vi "Testing Mode.vi"(8 "Filepath":path=path "D:/My Project/2019-2020/Magnetic Mareli UM/MM_UM/Project Setup/data/program seq/Program_280A.bin", 9 "FeedBack Channel":string[](array[string])=["fgdgfvcbc", "vnfhgjkn", "21354682"]) -> ()   [LabVIEW 2015]
uses:
  Control Button/Exit.ctl
  Control Button/Start.ctl
  Test  enqueue/AutoTest seq.ctl
  Test  enqueue/Auot Test selection.ctl
  <vilib>/Utility/error.llb/whitespace.ctl
  Galobal variable_TI.vi
  Project Setup/Globle Variable/GR_Servo.vi
  <vilib>/Utility/file.llb/Read Delimited Spreadsheet (string).vi
panel:
  out "Error  bit":bool
  out "reset":bool
  out "D-enqueue":T1
  in  "Report":bool
  in  "Tab Control":enum32{"Test", "Report"}(tab)
  in  "Boolean":bool=TRUE
  out "User Name":string
  in  "Table Control":string[][](table)
  out "Error Message":string
  out "Running Model":string
  out "Date time":string
  out "PCB Barcode":string
  out "Test Name":string
  in  "Tab Control 2":enum32{"Image", "Load and Lvdt"}(tab)
  out "2D Picture":picture
  out "Boolean 3":bool
  out "Waveform Graph":dbl[](graph)
  out "Error":bool
  in  "Exit":T2
  in  "Start 2":T3
  in  "Slide Servo Home Call":bool
  out "Servo Fault":bool
  in  "Servo Fault Reset":bool
  out "Actuator2(mm)":dbl format="%0.02f"
  out "Actuator1(mm)":dbl format="%0.02f"
  out "Load(N)":dbl format="%0.02f"
  out "Clip":T4
  in  "OK Counter":string
  in  "NG Counter":string
  out "Cycle Time(Sec)":i32
  out "Camera Result":bool
  in  "Report":i32(listbox)
  out "appended array":string[](array[string])
  in  "Sensor Feedback":T5(array[cluster])
  out "Start":bool
  in  "Cycle":i32
  in  "Home Call":bool
  out "DI":bool[](array[boolean])
  out "Current Date & Time":timestamp
  in  "Cycle Start Bit":bool
  in  "vi reference":refnum<vi>
  in  "Reset Ct.":bool
  out "error out":errorcluster
  in  "Tbl Refnum":refnum<vi>
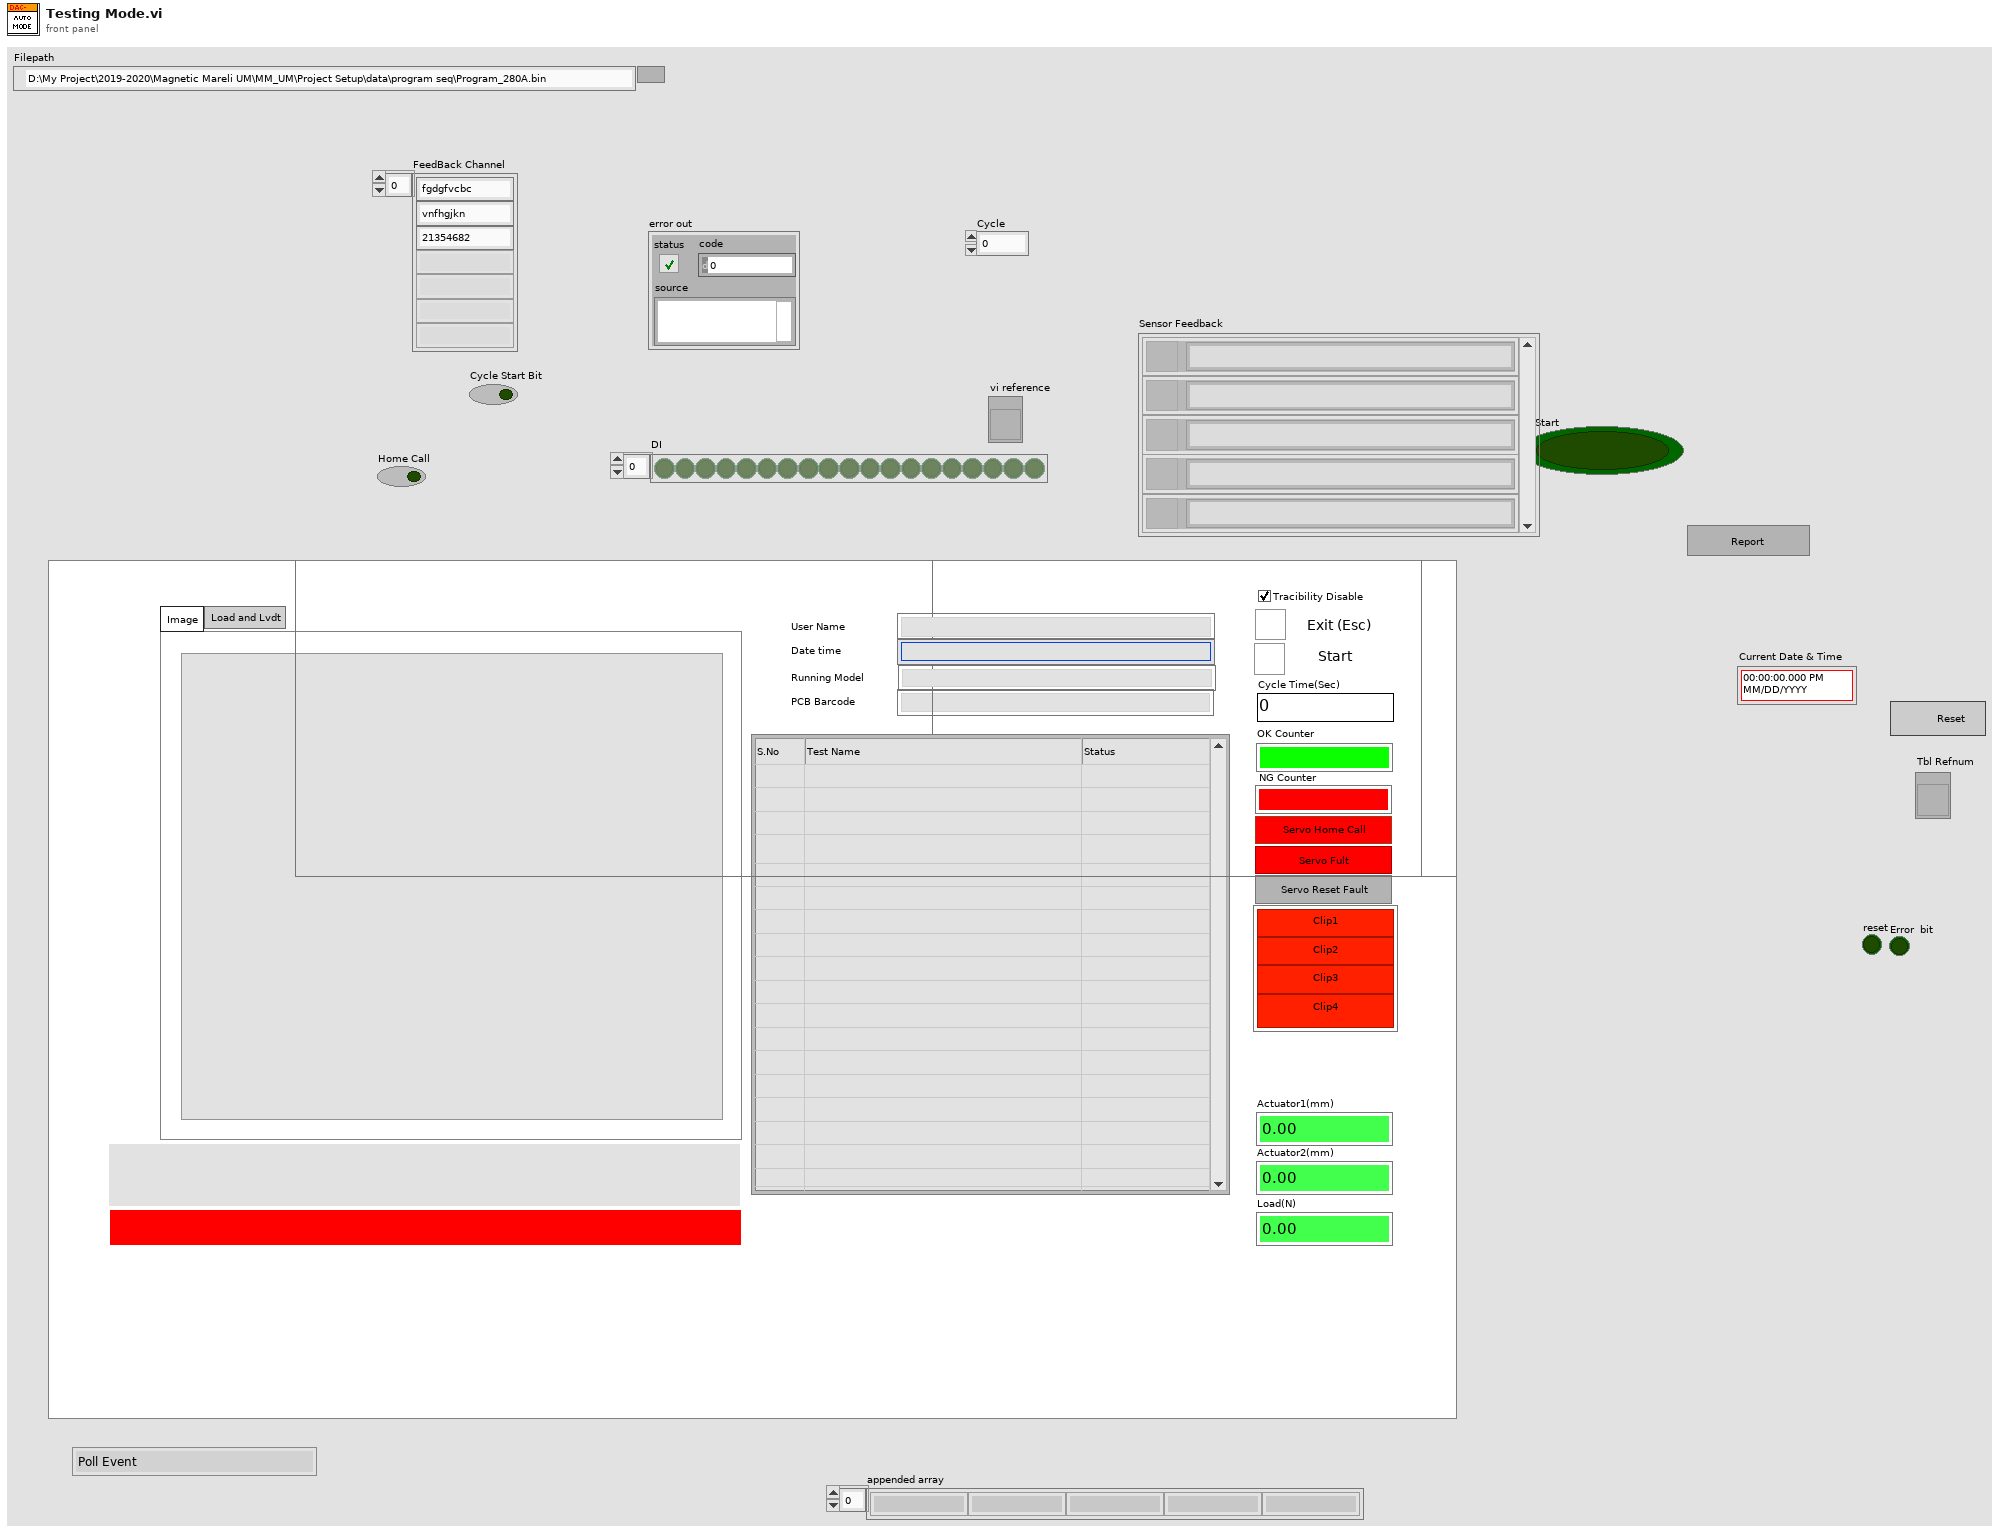
[diagram p1: front panel]
types:
  T1 = typedef "AutoTest seq.ctl" = enum16{"Poll Event", "Fixture 40 Deg up", "Program Seq", "Cylender Home", "Read Barcode", "Slide Servo send Cammand", "Slide Servo Home Call", "Camera Co-ordinate_1", "Camera Co-ordinate_2", "Result Save", "Error", "Exit"}
  T2 = typedef "Exit.ctl" = bool
  T3 = typedef "Start.ctl" = bool
  T4 = cluster{"Cllip-3 (AI12)":bool, "Cllip-4 (AI9)":bool, "Cllip-2(AI10)":bool, "Cllip-1 (AI9)":bool}
  T5 = cluster{"Sensor Name":string, "OK And NG":bool}[]
  T6 = cluster{"MIC ":refnum<visa-resource-name>, "baud rate MIC ":u32, "LCD ":refnum<visa-resource-name>, "baud rate_LCD":u32}
  T7 = typedef "Auot Test selection.ctl" = enum16{"Init", "Enqueue ", "Enqueue N", "Enqueue in stack", "Enqueue in stack N", "Dequeue", "Dequeue N", "Flush", "Release Queue"}
  T8 = cluster{"Item Name":string, "Item Status":bool, "Steps":cluster{"Channel Type":string, "Channels":string, "Wait/Poll (ms)":u32, "Parameter":u8, "STM-Speed":i32, "STM-Degree":u32, "Direction":u8}[]}[]
  T9 = cluster{"Actuator1(mm)":dbl, "Actuator2(mm)":dbl, "Load(N)":dbl, "Actuator1":bool, "Actuator2":bool, "Load":bool}
  T10 = enum16{"Part Clamp", "Part Unclamp", "Part Clamp Input Check", "Part Unclamp Input Check"}
  T11 = cluster{"Sr.No.":string, "Model Pass/Fail":string, "MIC Code":string, "Clip-1":string, "Clip-2":string, "Clip-3":string, "Clip-4":string, "Load Max":string, "Load Min":string, "Load Actual Value":string, "Actuator -1Min":string, "Actuator -1Max":string, "Actuator-1 Actual Value":string, "Actuator -2Min ":string, "Actuator -2Max ":string, "Actuator-2 Actual Value ":string, "Status":string}
  T12 = cluster{"No. Fail Coun t":string, "Rework Status Count 0\\1":string, "NA Count Max =3 ":string, "Testesd Count  0/1":string, "Error code":string}
  T13 = cluster{"Emergency_1":bool, "Reset_2":bool, "Home _3":bool, "Air Pressure_4":bool, "Safety Sensor_5":bool, "Safety Sensor_6":bool, "Slide Servo Home RS 26":bool, "LVDT UP RS":bool, "Servo Fault 27":bool, "Pressing UP RS 31":bool, "40 Deg. Down Fixture Rs":bool}
  T14 = typedef "whitespace.ctl" = u16
  T15 = cluster{"Load Max":string, "Load Min":string, "Actuator -1 Max":string, "Actuator -1 Min":string, "Actuator -2 Max":string, "Actuator -2 Min":string}
  T16 = cluster{"Sr.No.":string, "Model Name":string, "Date":string, "Time":string, "Model Pass/Fail":string, "MIC Code":string, "Clip-1":string, "Clip-2":string, "Clip-3":string, "Clip-4":string, "Load Max":string, "Load Min":string, "Load Actual Value":string, "Actuator -1Min":string, "Actuator -1Max":string, "Actuator-1 Actual Value":string, "Actuator -2Min ":string, "Actuator -2Max ":string, "Actuator-2 Actual Value ":string, "Status":string}
  T17 = cluster{"[0]":string, "[1]":string, "[2]":string, "[3]":string}
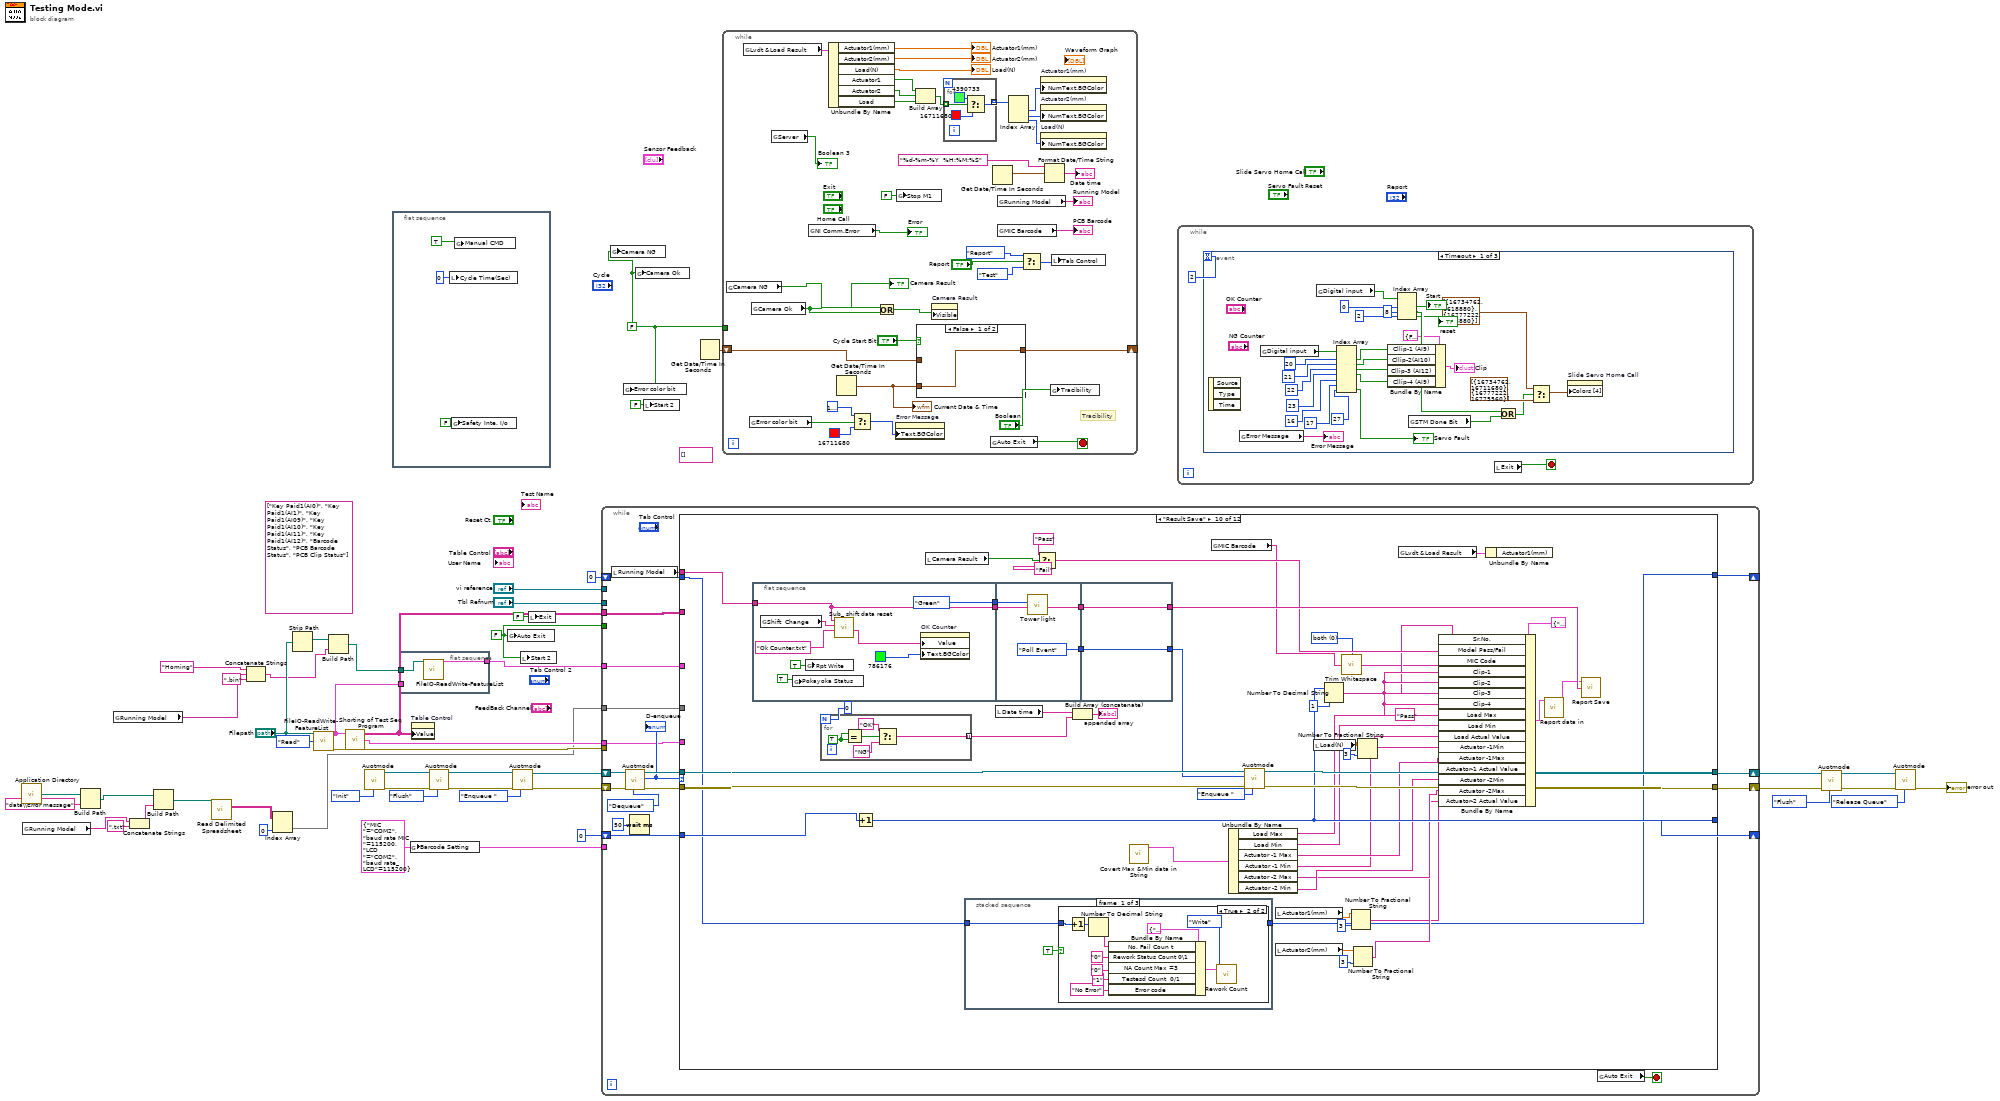
[diagram p0: block diagram]
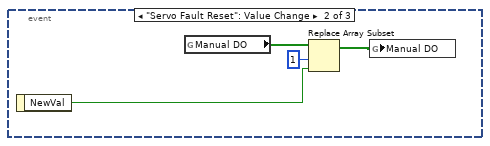
[diagram p2: hidden frame]
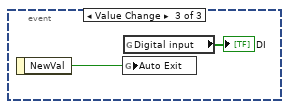
[diagram p3: hidden frame]
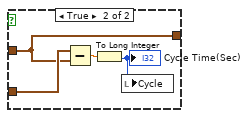
[diagram p4: hidden frame]
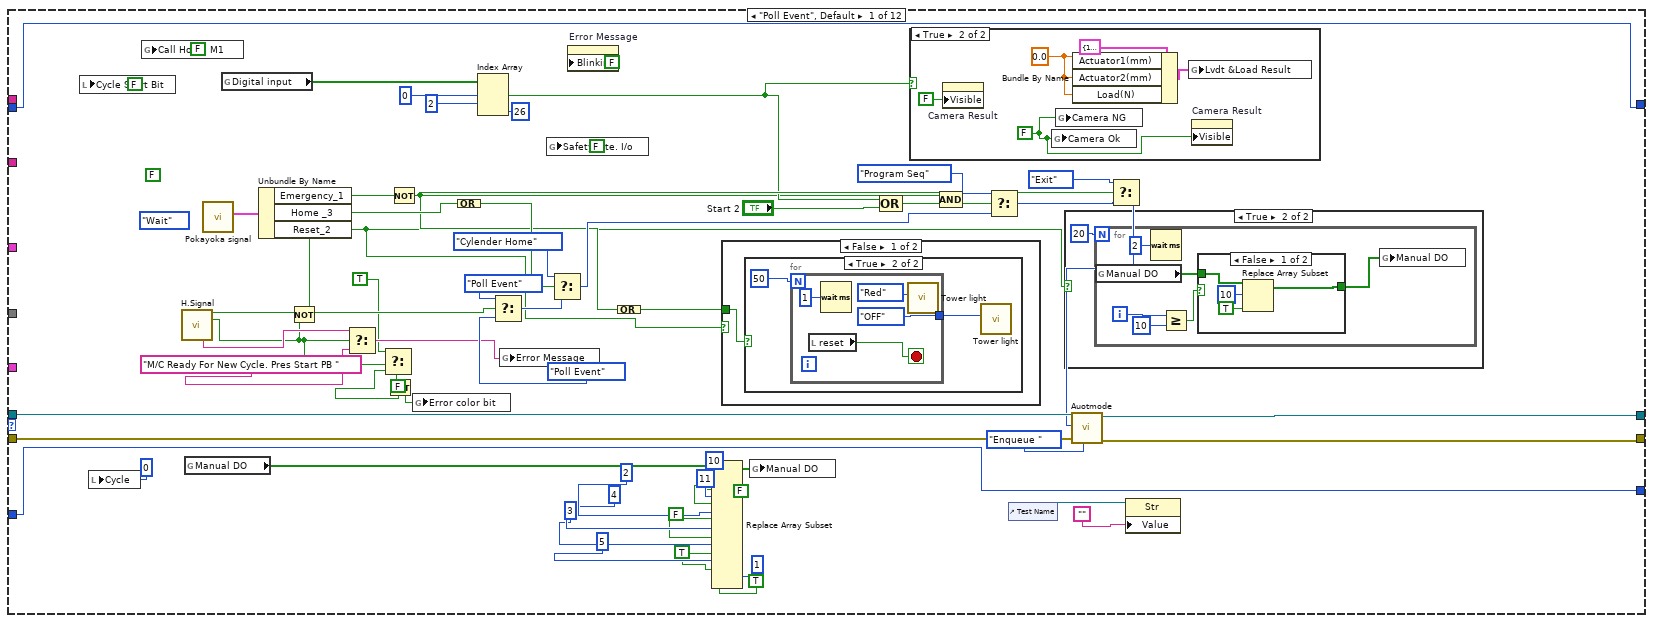
[diagram p5: hidden frame]
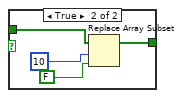
[diagram p7: hidden frame]
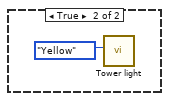
[diagram p10: hidden frame]
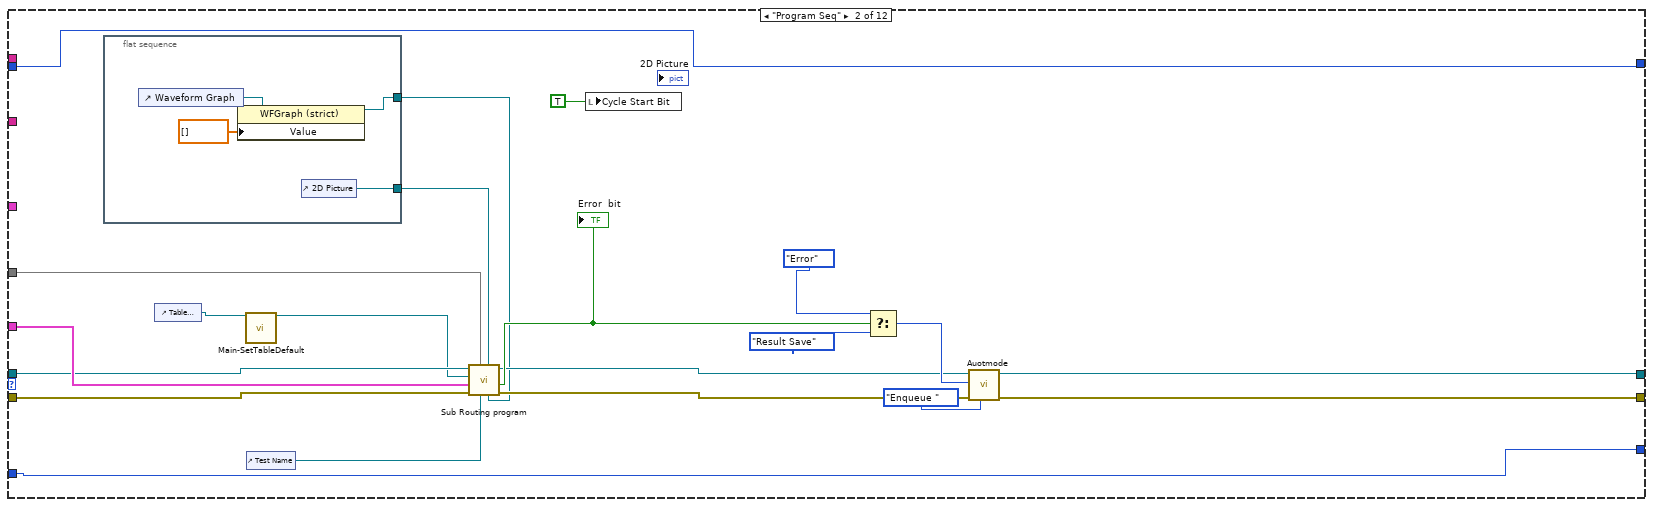
[diagram p11: hidden frame]
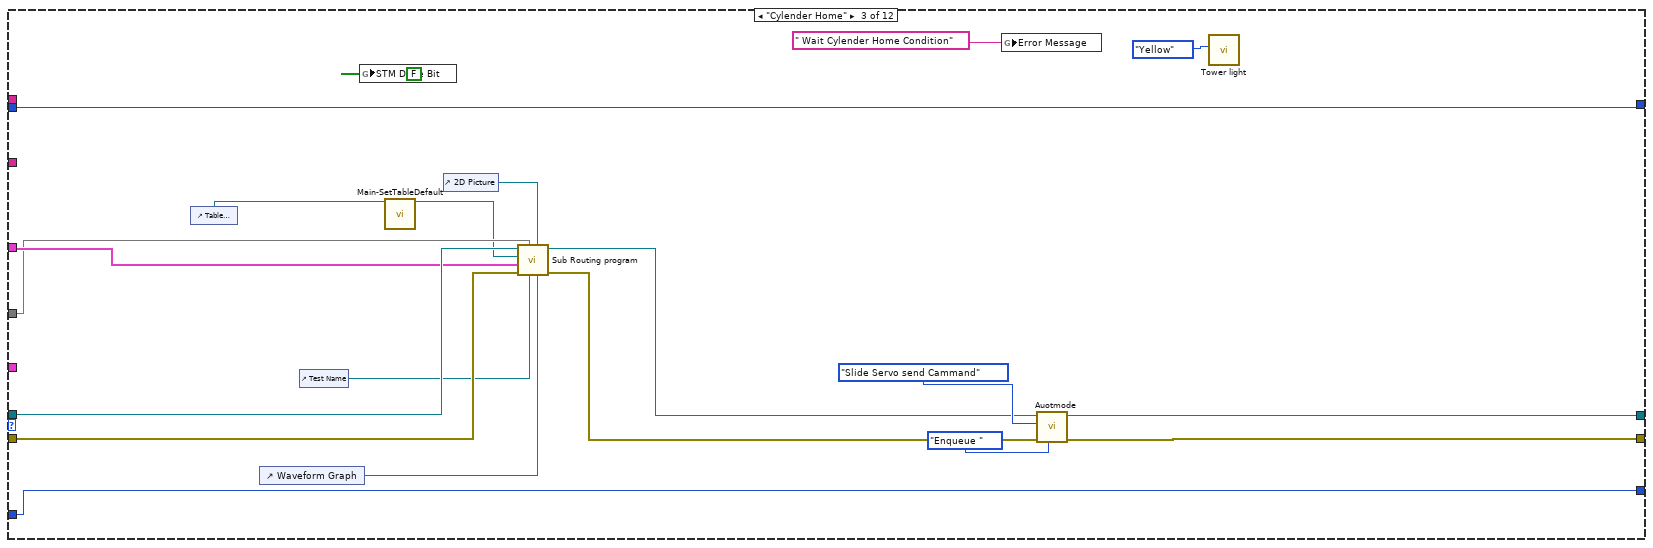
[diagram p12: hidden frame]
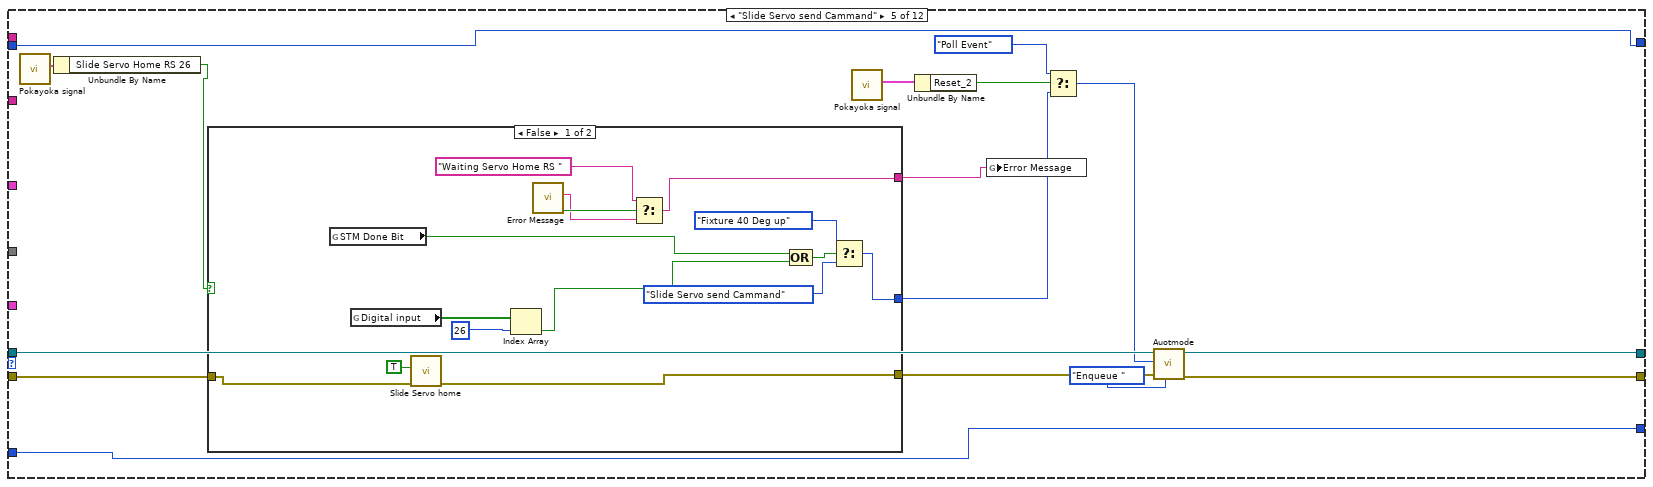
[diagram p14: hidden frame]
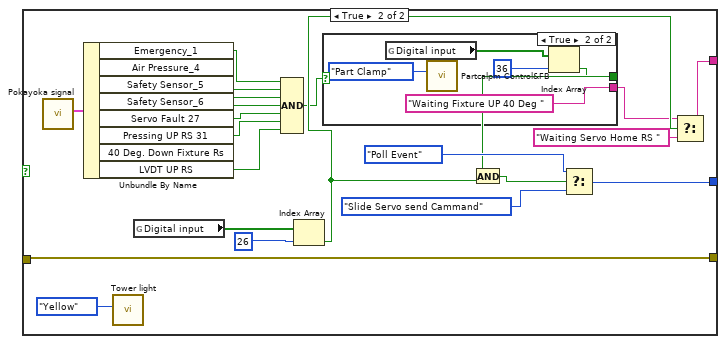
[diagram p15: hidden frame]
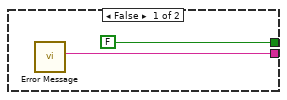
[diagram p16: hidden frame]
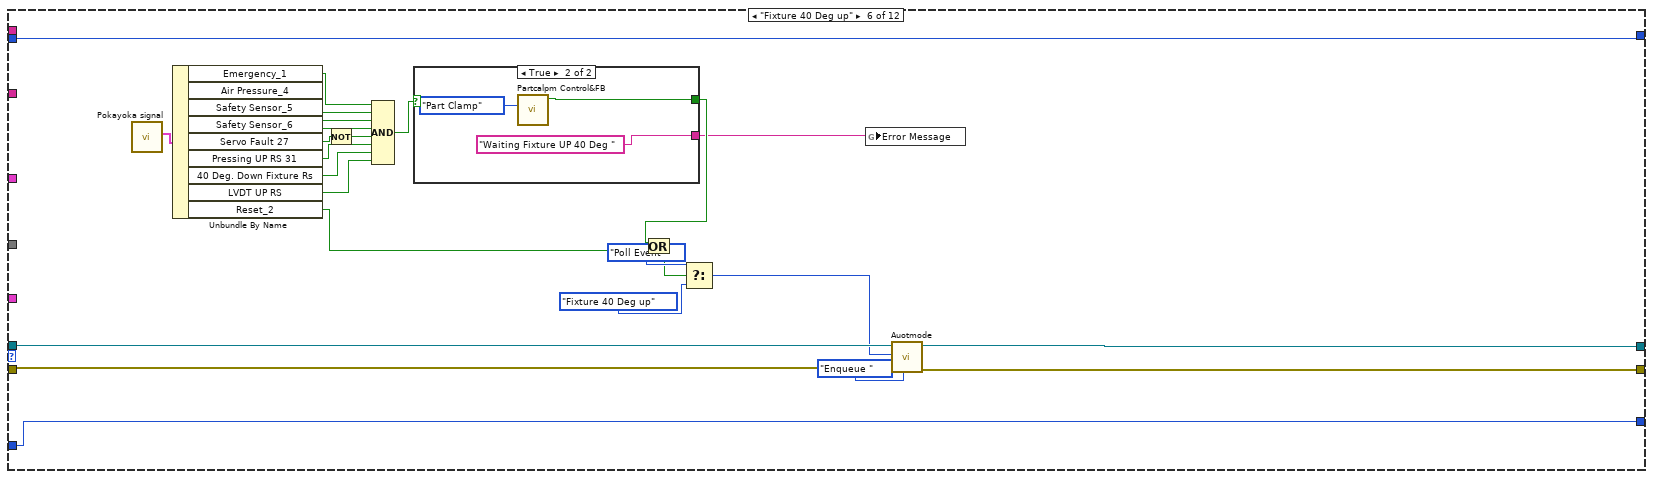
[diagram p17: hidden frame]
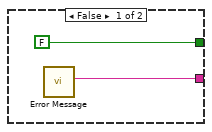
[diagram p18: hidden frame]
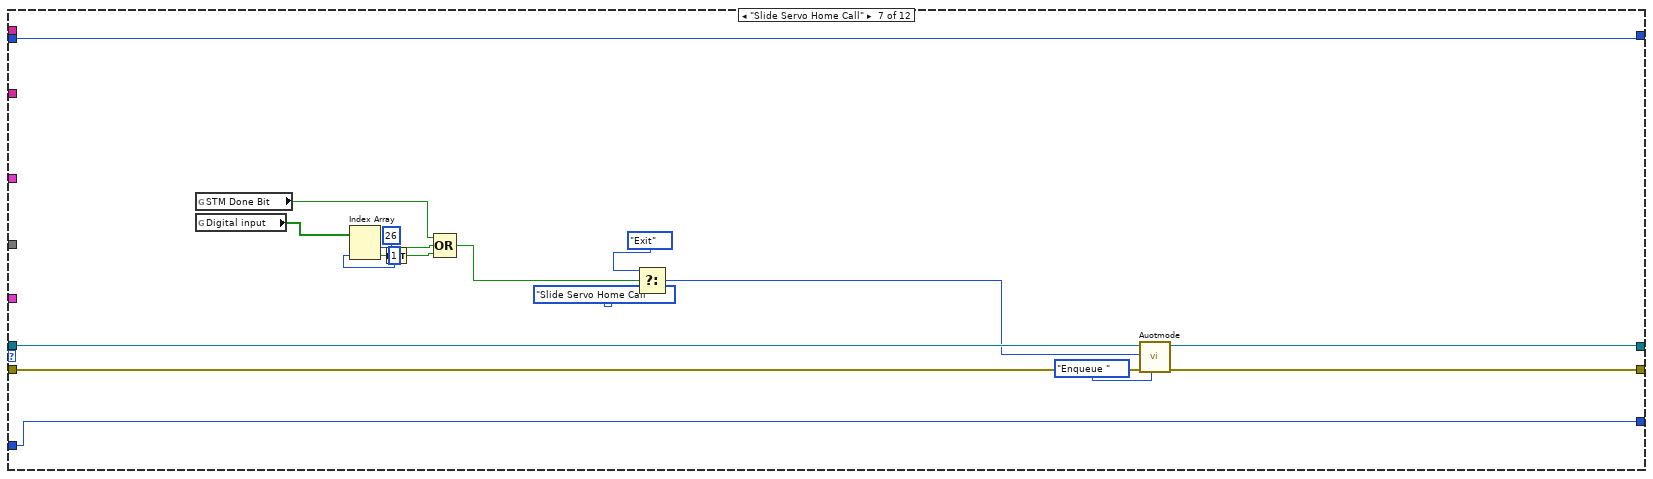
[diagram p19: hidden frame]
diagram:
  w18 = T6 {"MIC "="COM2", "baud rate MIC "=115200, "LCD "="COM2", "baud rate_LCD"=115200} ("Barcode Setting")
  (unwired) string[] ["Key Paid1(AI0)", "Key Paid1(AI1)", "Key Paid1(AI09)", "Key Paid1(AI10)", "Key Paid1(AI11)", "Key Paid1(AI12)", "Barcode Status", "PCB Barcode Status", "PCB Clip Status"] ("Error Name")
  (unwired) string[] []
  w3 = FALSE ("Servo Stop")
  w25 = FALSE ("Auto Exit")
  n1 = call <vilib>:"Application Directory.vi"() -> ("Application Directory"=w17:path)
  n2 = global read "Galobal variable_TI.vi" "Running Model"() -> (w14:string)
  n3 = Build Path(base path=w17, name or relative path="data\\Error message") -> (appended path=w15:path)
  n4 = global read "Galobal variable_TI.vi" "Running Model"() -> (w6:string)
  n5 = Concatenate Strings(w14, ".txt" ("string")) -> (w12:string)
  n6 = Build Path(base path=w15, name or relative path=w12) -> (appended path=w11:path)
  n7 = call-poly <vilib>:"Read Delimited Spreadsheet.vi"("file path (dialog if empty)"=w11) -> ("all rows"=w10:string[][])  [unwired: 9 in, 5 out]
  n8 = Concatenate Strings("Homing" ("name or relative path"), w6, ".bin" ("string")) -> (w4:string)
  n9 = Index Array(array=w10, index (col)=0 ("disabled index (col)")) -> (element=w8:string[])  [unwired: 1 in]
  n10 = Strip Path(path="Filepath") -> (stripped path=w22:path)  [unwired: 1 out]
  n11 = call "FileIO-ReadWrite-FeatureList.vi"("Filepath"="Filepath", "Read/Write"=enum16{"Read", "Write"}."Read") -> ("Feature List (Out)"=w20:T8, "Error Out"=w31:errorcluster)  [unwired: 12 in]
  n12 = Build Path(base path=w22, name or relative path=w4) -> (appended path=w21:path)
  n13 = call "Shorting of Test Seq Program.vi"("Feature List (Out)"=w20) -> ("Feature Step Enable"=w27:T8, "Feature Name"=w26:string[][])  [unwired: 3 in]
  n14 = call "Auotmode.vi"("Enum Selection"=Auot_Test_selection."Init") -> ("error out"=w43:errorcluster, "queue Out"=w41:refnum<queue>)  [unwired: 7 in, 1 out]
  n15 = flat-sequence {
    frame #0 {
      n16 = local write "Cycle Time(Sec)"(0 ("Cycle Time(Sec)")) -> ()
      n17 = global write "Galobal variable_TI.vi" "Safety Inte. I/o"(FALSE ("Safety Inte. I/o")) -> ()
      n18 = global write "Galobal variable_TI.vi" "Manual CMD"(TRUE ("Manual CMD")) -> ()
    }
  }
  n19 = flat-sequence {
    tunnel: w21 -> [w54]
    tunnel: w20 -> [_]
    tunnel: [w53] -> w19
    frame #0 {
      n20 = call "FileIO-ReadWrite-FeatureList.vi"("Filepath"=w54) -> ("Feature List (Out)"=w53:T8)  [unwired: 13 in, 1 out]
    }
  }
  n21 = global write "Galobal variable_TI.vi" "Barcode Setting"(w18) -> ()
  n22 = property on="Table Control" class="Tbl (strict)"("Value"=w26) -> ()  [unwired: 2 in, 2 out]
  n23 = call "Auotmode.vi"("Enum Selection"=Auot_Test_selection."Flush", "Error In"=w43, "queue in"=w41) -> ("error out"=w42:errorcluster, "queue Out"=w40:refnum<queue>)  [unwired: 5 in, 1 out]
  n24 = global write "Galobal variable_TI.vi" "Auto Exit"(w25) -> ()
  n25 = call "Auotmode.vi"("Enum Selection"=Auot_Test_selection."Enqueue ", "Error In"=w42, "queue in"=w40) -> ("error out"=w47:errorcluster, "queue Out"=w29:refnum<queue>)  [unwired: 5 in, 1 out]
  n26 = local write "Start 2"(w25) -> ()
  n27 = local write "Exit"(T2 FALSE ("Exit")) -> ()
  n28 = while {
    tunnel: "vi reference" -> [_]
    tunnel: "Tbl Refnum" -> [_]
    tunnel: w27 -> [w66]
    tunnel: w31 -> [_]
    tunnel: w8 -> [w67]
    shift-right: [w70] -> w34
    shift-left: w29 -> [w63]
    shift-right: [w62] -> w28
    shift-left: w47 -> [w72]
    tunnel: w25 -> [_]
    tunnel: w26 -> [w61]
    tunnel: w19 -> [w59]
    tunnel: w18 -> [_]
    shift-right: [w57] -> _
    shift-left: u32 0 ("milliseconds to wait") -> [w58]
    shift-right: [w55] -> _
    shift-left: u32 0 ("milliseconds to wait") -> [w56]
    stop <- w65 stop-if-true
    n29 = local read "Running Model"() -> (w60:string)
    n30 = call "Auotmode.vi"("Enum Selection"=Auot_Test_selection."Dequeue", "Error In"=w72, "queue in"=w63) -> ("error out"=w69:errorcluster, "D-enqueue"=w68:T1, "queue Out"=w71:refnum<queue>)  [unwired: 5 in]
    "D-enqueue" <- w68
    n31 = Wait (ms)(milliseconds to wait=u32 50) -> ()  [unwired: 1 out]
    n32 = case shown="\"Result Save\"" w68 {
      tunnel: w71 -> [w134 w172 w204 w211 w222 w284 w316 w323 w327 w376 w432 w544]
      tunnel: [w132 w179 w206 w211 w226 w283 w317 w323 w327 w374 w431 w545] -> w70
      tunnel: w69 -> [w133 w174 w203 w210 w224 w282 w315 w322 w326 w375 w430 w546]
      tunnel: [w131 w178 w205 w210 w225 w281 w318 w322 w326 w373 w429 w546] -> w62
      tunnel: w66 -> [_ w175 _ _ _ _ _ _ _ _ _ _]
      tunnel: w67 -> [_ w176 w201 _ _ _ _ _ _ _ _ _]
      tunnel: w61 -> [_ _ _ _ _ _ _ _ _ _ _ _]
      tunnel: w60 -> [_ _ _ _ _ _ _ _ _ w372 w416 _]
      tunnel: w59 -> [_ _ w202 _ _ _ _ _ _ _ _ _]
      tunnel: w58 -> [w75 w164 w189 w209 w213 w273 w303 w321 w325 w355 w415 w530]
      tunnel: [w75 w164 w189 w209 w213 w273 w303 w321 w325 w354 w415 w530] -> w57
      tunnel: w56 -> [w74 w163 w188 w208 w212 w272 w302 w320 w324 w329 w412 w529]
      tunnel: [w74 w163 w188 w208 w212 w272 w302 w320 w324 w328 w411 w529] -> w55
      frame "Poll Event", Default {
        w79 = TRUE ("new element/subarray")
        w80 = FALSE ("new element/subarray")
        w98 = FALSE ("new element/subarray")
        (unwired) enum16{"Wait", "Ionizer On", "Ionizer off"}."Wait" ("Enum")
        (unwired) FALSE ("Ionizer cnf")
        n33 = local write "Cycle Start Bit"(FALSE ("Cycle Start Bit")) -> ()
        n34 = local write "Cycle"(0 ("Cycle")) -> ()
        n35 = global write "Galobal variable_TI.vi" "Call Home M1"(FALSE ("Call Home M1")) -> ()
        n36 = call "H.Signal.vi"() -> ("Slide servo home RS"=w119:bool, "HI Bit Auto"=w88:bool, "Message"=w95:string)  [unwired: 10 in, 3 out]
        n37 = global read "Galobal variable_TI.vi" "Manual DO"() -> (w86:bool[])
        n38 = call "Pokayoka signal.vi"() -> ("output cluster"=w113:T13)  [unwired: 10 in, 1 out]
        n39 = global read "Galobal variable_TI.vi" "Digital input"() -> (w129:bool[])
        n40 = Unbundle By Name(w113) -> ("Emergency_1"=w112:bool, "Home _3"=w103:bool, "Reset_2"=w96:bool)
        n41 = Not(x=w88) -> (.not. x?=w87:bool)
        n42 = Select(t=w95, s=w88, f="M/C Ready For New Cycle. Pres Start PB ") -> (s? t:f=w108:string)
        n43 = Select(t=TRUE, s=w88, f=FALSE) -> (s? t:f=w92:bool)
        n44 = Not(x=w92) -> (.not. x?=w91:bool)
        n45 = Not(x=w112) -> (.not. x?=w102:bool)
        n46 = global write "Galobal variable_TI.vi" "Error color bit"(w91) -> ()
        n47 = Compound Arithmetic op=OR(w103) -> (w125:bool)
        n48 = Index Array(array=w129, index #1=0 ("index"), index #2=2 ("index"), index #3=26 ("index")) -> (element #1=w97:bool)  [unwired: 2 out]
        n49 = Select(t=AutoTest_seq."Poll Event" ("Enqueue"), s=w119, f=AutoTest_seq."Poll Event") -> (s? t:f=w123:T1)
        n50 = global write "GR_Servo.vi" "Error Message"(w108) -> ()
        n51 = global write "Galobal variable_TI.vi" "Safety Inte. I/o"(FALSE ("Safety Inte. I/o")) -> ()
        n52 = Select(t=AutoTest_seq."Cylender Home" ("Enqueue"), s=w125, f=w123) -> (s? t:f=w111:T1)
        n53 = property on="Error Message" class="Str"("Blinking"=FALSE) -> ()  [unwired: 2 in, 2 out]
        n54 = Compound Arithmetic op=OR(w102) -> (w107:bool)
        n55 = Replace Array Subset(array=w86, new element #1=w98, index #1=10 ("index"), new element #2=w98, index #2=11 ("index"), new element #3=w80, index #3=2 ("index"), new element #4=w80, index #4=4 ("index"), new element #5=w79, index #5=3 ("index"), new element #6=w79, index #6=5 ("index"), new element #7=TRUE ("new element/subarray"), index #7=1 ("index")) -> (w101:bool[])
        n56 = case shown="False" w96 {
          tunnel: w107 -> [w155 _]
          frame False {
            n57 = case shown="True" w155 {
              frame False {
              }
              frame True {
                n58 = for {
                  N: 50 -> [_]
                  tunnel: [enum16{"Green", "Red", "Yellow", "OFF"}."OFF" ("Enum")] -> w156
                  stop <- w158 stop-if-true
                  n59 = local read "reset"() -> (w158:bool)
                  n60 = Wait (ms)(milliseconds to wait=u32 1) -> ()  [unwired: 1 out]
                  n61 = call "Tower light.vi"("Enum"=enum16{"Green", "Red", "Yellow"}."Red") -> ()  [unwired: 11 in]
                }
                n62 = call "Tower light.vi"("Enum"=w156) -> ()  [unwired: 11 in]
              }
            }
          }
          frame True {
            n63 = call "Tower light.vi"("Enum"=enum16{"Green", "Red", "Yellow"}."Yellow") -> ()  [unwired: 11 in]
          }
        }
        n64 = global write "Galobal variable_TI.vi" "Manual DO"(w101) -> ()
        n65 = Compound Arithmetic op=OR(w97, "Start 2") -> (w117:T3)
        n66 = case shown="True" w97 {
          frame False {
          }
          frame True {
            w150 = 0.0
            w153 = FALSE
            n67 = property on="Camera Result" class="Bool (strict)"("Visible"=FALSE) -> ()  [unwired: 2 in, 2 out]
            n68 = global write "Galobal variable_TI.vi" "Camera Ok"(w153) -> ()
            n69 = global write "Galobal variable_TI.vi" "Camera NG"(w153) -> ()
            n70 = Bundle By Name(cluster=T9 {"Actuator1(mm)"=1.6341840742039335, "Actuator2(mm)"=1.8426400447473008, "Load(N)"=41.278042038610465, "Actuator1"=TRUE, "Actuator2"=TRUE, "Load"=TRUE} ("Lvdt &Load Result"), "Actuator1(mm)"=w150, "Actuator2(mm)"=w150, "Load(N)"=w150) -> (w151:T9)
            n71 = global write "Galobal variable_TI.vi" "Lvdt &Load Result"(w151) -> ()
            n72 = property on="Camera Result" class="Bool (strict)"("Visible"=w153) -> ()  [unwired: 2 in, 2 out]
          }
        }
        n73 = Compound Arithmetic op=AND(w87, w117) -> (w89:T3)
        n74 = Select(t=AutoTest_seq."Program Seq" ("Enqueue"), s=w89, f=w111) -> (s? t:f=w105:T1)
        n75 = control-ref of="Test Name"() -> (w110:refnum<vi>)
        n76 = case shown="True" w96 {
          frame False {
          }
          frame True {
            n77 = for {
              N: 20 -> [_]
              i -> [w141]
              n78 = global read "Galobal variable_TI.vi" "Manual DO"() -> (w138:bool[])
              n79 = Wait (ms)(milliseconds to wait=u32 2) -> ()  [unwired: 1 out]
              n80 = Greater Or Equal?(x=w141, y=10) -> (x >= y?=w139:bool)
              n81 = case shown="False" w139 {
                tunnel: w138 -> [w145 w147]
                tunnel: [w142 w146] -> w137
                frame False {
                  n82 = Replace Array Subset(array=w145, new element=TRUE ("new element/subarray"), index=10) -> (w142:bool[])
                }
                frame True {
                  n83 = Replace Array Subset(array=w147, new element=FALSE ("new element/subarray"), index=10) -> (w146:bool[])
                }
              }
              n84 = global write "Galobal variable_TI.vi" "Manual DO"(w137) -> ()
            }
          }
        }
        n85 = Select(t=AutoTest_seq."Exit" ("Enqueue"), s=w102, f=w105) -> (s? t:f=w106:T1)
        n86 = call "Auotmode.vi"("Enum Selection"=Auot_Test_selection."Enqueue ", "Error In"=w133, "Enqueue"=w106, "queue in"=w134) -> ("error out"=w131:errorcluster, "queue Out"=w132:refnum<queue>)  [unwired: 4 in, 1 out]
        n87 = property class="Str"(reference=w110, "Value"="") -> ()  [unwired: 1 in, 2 out]
      }
      frame "Program Seq" {
        n88 = flat-sequence {
          tunnel: [w187] -> w169
          tunnel: [w184] -> w165
          frame #0 {
            n89 = control-ref of="Waveform Graph"() -> (w186:refnum<vi>)
            n90 = property class="WFGraph (strict)"(reference=w186, "Value"=dbl[] []) -> (reference out=w184:refnum<vi>)  [unwired: 1 in, 1 out]
            n91 = control-ref of="2D Picture"() -> (w187:refnum<vi>)
          }
        }
        n92 = control-ref of="Table Control"() -> (w168:refnum<vi>)
        n93 = call "Main-SetTableDefault.vi"("Table (In)"=w168) -> ("Table (Out)"=w167:refnum<vi>)  [unwired: 13 in, 1 out]
        n94 = control-ref of="Test Name"() -> (w170:refnum<vi>)
        n95 = call "Sub Routing program.vi"("Load Graph"=w165, "Image"=w169, "Test Name"=w170, "FeedBack Channel"=w176, "error in (no error)"=w174, "Feature Step Enable"=w175, "Table"=w167, "queue Out in"=w172) -> ("error out"=w173:errorcluster, "Error"=w177:bool, "Queue out"=w171:refnum<queue>)  [unwired: 1 out]
        "Error  bit" <- w177
        n96 = local write "Cycle Start Bit"(TRUE ("Cycle Start Bit")) -> ()
        n97 = Select(t=AutoTest_seq."Error" ("Enqueue"), s=w177, f=AutoTest_seq."Result Save" ("Enqueue")) -> (s? t:f=w180:T1)
        n98 = call "Auotmode.vi"("Enum Selection"=Auot_Test_selection."Enqueue ", "Error In"=w173, "Enqueue"=w180, "queue in"=w171) -> ("error out"=w178:errorcluster, "queue Out"=w179:refnum<queue>)  [unwired: 4 in, 1 out]
      }
      frame "Cylender Home" {
        n99 = control-ref of="Table Control"() -> (w198:refnum<vi>)
        n100 = control-ref of="Waveform Graph"() -> (w191:refnum<vi>)
        n101 = control-ref of="Test Name"() -> (w200:refnum<vi>)
        n102 = global write "Galobal variable_TI.vi" "STM Done Bit"(FALSE ("STM Done Bit")) -> ()
        n103 = call "Main-SetTableDefault.vi"("Table (In)"=w198) -> ("Table (Out)"=w192:refnum<vi>)  [unwired: 13 in, 1 out]
        n104 = control-ref of="2D Picture"() -> (w193:refnum<vi>)
        n105 = call "Sub Routing program.vi"("Load Graph"=w191, "Image"=w193, "Test Name"=w200, "FeedBack Channel"=w201, "error in (no error)"=w203, "Feature Step Enable"=w202, "Table"=w192, "queue Out in"=w204) -> ("error out"=w195:errorcluster, "Queue out"=w194:refnum<queue>)  [unwired: 2 out]
        n106 = global write "GR_Servo.vi" "Error Message"(" Wait Cylender Home Condition") -> ()
        n107 = call "Auotmode.vi"("Enum Selection"=Auot_Test_selection."Enqueue ", "Error In"=w195, "Enqueue"=AutoTest_seq."Slide Servo send Cammand", "queue in"=w194) -> ("error out"=w205:errorcluster, "queue Out"=w206:refnum<queue>)  [unwired: 4 in, 1 out]
        n108 = call "Tower light.vi"("Enum"=enum16{"Green", "Red", "Yellow"}."Yellow") -> ()  [unwired: 11 in]
      }
      frame "Read Barcode" {
      }
      frame "Slide Servo send Cammand" {
        n109 = call "Pokayoka signal.vi"() -> ("output cluster"=w221:T13)  [unwired: 10 in, 1 out]
        n110 = Unbundle By Name(w221) -> ("Slide Servo Home RS 26"=w220:bool)
        n111 = case shown="False" w220 {
          tunnel: w224 -> [w242 w264]
          tunnel: [w241 w264] -> w223
          tunnel: [w236 w261] -> w215
          tunnel: [w228 w253] -> w219
          frame False {
            n112 = global read "Galobal variable_TI.vi" "STM Done Bit"() -> (w239:bool)
            n113 = global read "Galobal variable_TI.vi" "Digital input"() -> (w234:bool[])
            n114 = call "Slide Servo home.vi"("error in"=w242, "NewVal"=TRUE) -> ("error out"=w241:errorcluster)  [unwired: 9 in]
            n115 = Index Array(array=w234, index=26) -> (element=w232:bool)
            n116 = call "Error Message.vi"() -> ("logical AND"=w231:bool, "Error"=w229:string)  [unwired: 10 in]
            n117 = Select(t="Waiting Servo Home RS " ("f"), s=w231, f=w229) -> (s? t:f=w228:string)
            n118 = Compound Arithmetic op=OR(w239, w232) -> (w235:bool)
            n119 = Select(t=AutoTest_seq."Fixture 40 Deg up" ("Enqueue"), s=w235, f=AutoTest_seq."Slide Servo send Cammand" ("Enqueue")) -> (s? t:f=w236:T1)
          }
          frame True {
            n120 = call "Pokayoka signal.vi"() -> ("output cluster"=w246:T13)  [unwired: 10 in, 1 out]
            n121 = Unbundle By Name(w246) -> ("Emergency_1"=w251:bool, "Air Pressure_4"=w247:bool, "Safety Sensor_5"=w248:bool, "Safety Sensor_6"=w249:bool, "Servo Fault 27"=w250:bool, "Pressing UP RS 31"=w252:bool, "LVDT UP RS"=w244:bool)  [unwired: 1 out]
            n122 = call "Tower light.vi"("Enum"=enum16{"Green", "Red", "Yellow"}."Yellow") -> ()  [unwired: 11 in]
            n123 = global read "Galobal variable_TI.vi" "Digital input"() -> (w260:bool[])
            n124 = Compound Arithmetic op=AND(w251, w247, w248, w249, w250, w252, w244) -> (w245:bool)
            n125 = Index Array(array=w260, index=26) -> (element=w254:bool)
            n126 = case shown="True" w245 {
              tunnel: [FALSE ("Part Clamp Feedback") w267] -> w257
              tunnel: [w265 "Waiting Fixture UP 40 Deg " ("f")] -> w243
              frame False {
                n127 = call "Error Message.vi"() -> ("Error"=w265:string)  [unwired: 10 in, 1 out]
              }
              frame True {
                n128 = global read "Galobal variable_TI.vi" "Digital input"() -> (w268:bool[])
                n129 = call "Partcalpm Control&FB.vi"("Enum"=T10."Part Clamp") -> ()  [unwired: 9 in, 2 out]
                n130 = Index Array(array=w268, index=36) -> (element=w267:bool)
              }
            }
            n131 = And(x=w257, y=w254) -> (x .and. y?=w256:bool)
            n132 = Select(t=AutoTest_seq."Poll Event" ("Enqueue"), s=w256, f=AutoTest_seq."Slide Servo send Cammand" ("Enqueue")) -> (s? t:f=w261:T1)
            n133 = Select(t=w243, s=w254, f="Waiting Servo Home RS ") -> (s? t:f=w253:string)
          }
        }
        n134 = call "Pokayoka signal.vi"() -> ("output cluster"=w218:T13)  [unwired: 10 in, 1 out]
        n135 = Unbundle By Name(w218) -> ("Reset_2"=w217:bool)
        n136 = global write "GR_Servo.vi" "Error Message"(w219) -> ()
        n137 = Select(t=AutoTest_seq."Poll Event" ("Enqueue"), s=w217, f=w215) -> (s? t:f=w214:T1)
        n138 = call "Auotmode.vi"("Enum Selection"=Auot_Test_selection."Enqueue ", "Error In"=w223, "Enqueue"=w214, "queue in"=w222) -> ("error out"=w225:errorcluster, "queue Out"=w226:refnum<queue>)  [unwired: 4 in, 1 out]
      }
      frame "Fixture 40 Deg up" {
        n139 = call "Pokayoka signal.vi"() -> ("output cluster"=w287:T13)  [unwired: 10 in, 1 out]
        n140 = Unbundle By Name(w287) -> ("Emergency_1"=w292:bool, "Air Pressure_4"=w288:bool, "Safety Sensor_5"=w289:bool, "Safety Sensor_6"=w290:bool, "Servo Fault 27"=w291:bool, "Pressing UP RS 31"=w293:bool, "40 Deg. Down Fixture Rs"=w294:bool, "LVDT UP RS"=w295:bool, "Reset_2"=w274:bool)
        n141 = Not(x=w291) -> (.not. x?=w296:bool)
        n142 = Compound Arithmetic op=AND(w292, w288, w289, w290, w296, w293, w294, w295) -> (w286:bool)
        n143 = case shown="True" w286 {
          tunnel: [FALSE ("Part Clamp Feedback") w301] -> w280
          tunnel: [w297 "Waiting Fixture UP 40 Deg " ("f")] -> w279
          frame False {
            n144 = call "Error Message.vi"() -> ("Error"=w297:string)  [unwired: 10 in, 1 out]
          }
          frame True {
            n145 = call "Partcalpm Control&FB.vi"("Enum"=T10."Part Clamp") -> ("Part Clamp Feedback"=w301:bool)  [unwired: 9 in, 1 out]
          }
        }
        n146 = Or(x=w280, y=w274) -> (x .or. y?=w275:bool)
        n147 = Select(t=AutoTest_seq."Poll Event" ("Enqueue"), s=w275, f=AutoTest_seq."Fixture 40 Deg up" ("Enqueue")) -> (s? t:f=w276:T1)
        n148 = global write "GR_Servo.vi" "Error Message"(w279) -> ()
        n149 = call "Auotmode.vi"("Enum Selection"=Auot_Test_selection."Enqueue ", "Error In"=w282, "Enqueue"=w276, "queue in"=w284) -> ("error out"=w281:errorcluster, "queue Out"=w283:refnum<queue>)  [unwired: 4 in, 1 out]
      }
      frame "Slide Servo Home Call" {
        n150 = global read "Galobal variable_TI.vi" "STM Done Bit"() -> (w309:bool)
        n151 = global read "Galobal variable_TI.vi" "Digital input"() -> (w307:bool[])
        n152 = Index Array(array=w307, index #1=26 ("index"), index #2=1 ("index")) -> (element #1=w308:bool, element #2=w305:bool)
        n153 = Not(x=w305) -> (.not. x?=w304:bool)
        n154 = Compound Arithmetic op=OR(w309, w308, w304) -> (w311:bool)
        n155 = Select(t=AutoTest_seq."Exit" ("Enqueue"), s=w311, f=AutoTest_seq."Slide Servo Home Call" ("Enqueue")) -> (s? t:f=w314:T1)
        n156 = call "Auotmode.vi"("Enum Selection"=Auot_Test_selection."Enqueue ", "Error In"=w315, "Enqueue"=w314, "queue in"=w316) -> ("error out"=w318:errorcluster, "queue Out"=w317:refnum<queue>)  [unwired: 4 in, 1 out]
      }
      frame "Camera Co-ordinate_1" {
      }
      frame "Camera Co-ordinate_2" {
      }
      frame "Result Save" {
        w349 = T14 0 items=["both", "start of string", "end of string"] ("location (both)")
        w356 = "Pass" ("Status")
        n157 = flat-sequence {
          tunnel: w372 -> [w401]
          tunnel: [enum16{"Green", "Red", "Yellow"}."Green" ("Enum")] -> w371
          tunnel: [w401] -> w362
          tunnel: w371 -> [w408]
          tunnel: [AutoTest_seq."Poll Event" ("Enqueue")] -> w369
          tunnel: [w406] -> w363
          tunnel: w362 -> [w406]
          tunnel: [w410] -> w370
          tunnel: w369 -> [w410]
          tunnel: [w409] -> w364
          tunnel: w363 -> [w409]
          frame #0 {
            n158 = global read "Galobal variable_TI.vi" "Shift  Change"() -> (w398:string)
            n159 = global write "Galobal variable_TI.vi" "Pokayoka Status"(TRUE ("Rpt Read")) -> ()
            n160 = global write "Galobal variable_TI.vi" "Rpt Write"(TRUE ("Rpt Read")) -> ()
            n161 = call "Sub_ shift data reset.vi"("Serial no"="Ok Counter.txt" ("File Name"), "Shift"=w398, "Model"=w401) -> ("Serial no"=w404:string)  [unwired: 6 in, 1 out]
            n162 = property on="OK Counter" class="Str"("Value"=w404, "Text.BGColor"=u32 786176 ("Color Box")) -> ()  [unwired: 2 in, 2 out]
          }
          frame #1 {
            n163 = call "Tower light.vi"("Enum"=w408) -> ()  [unwired: 11 in]
          }
          frame #2 {
          }
        }
        n164 = for {
          N: 0 -> [_]
          tunnel: [w394] -> w367 mode=indexing
          w393 = TRUE ("y")
          n165 = Equal?(x=w393, y=w393) -> (x = y?=w397:bool)
          n166 = Select(t="OK", s=w397, f="NG") -> (s? t:f=w394:string)
        }
        n167 = Increment(x=w355) -> (x+1=w354:u32)
        n168 = local read "Camera Result"() -> (w360:bool)
        n169 = stacked-sequence {
          tunnel: w329 -> [w379 _ _]
          tunnel: [_ _ u32 0 ("milliseconds to wait")] -> w328
          frame #0 {
            n170 = case shown="True" TRUE {
              tunnel: w379 -> [_ w385]
              frame False {
              }
              frame True {
                n171 = Increment(x=w385) -> (x+1=w381:u32)
                n172 = Number To Decimal String(number=w381) -> (decimal integer string=w384:string)  [unwired: 1 in]
                n173 = Bundle By Name(cluster=T12 {"No. Fail Coun t"="", "Rework Status Count 0\\1"="", "NA Count Max =3 "="", "Testesd Count  0/1"="", "Error code"=""} ("Count For Rework"), "No. Fail Coun t"=w384, "Rework Status Count 0\\1"="0" ("Rework Status Count 0\\1"), "NA Count Max =3"="0", "Testesd Count  0/1"="1", "Error code"="No Error") -> (w383:T12)
                n174 = call "Rework Count.vi"("Read /Write"=enum16{"Write", "Read"}."Write", "Count For Rework"=w383) -> ()  [unwired: 8 in, 2 out]
              }
            }
          }
          frame #1 {
            n175 = Wait (ms)(milliseconds to wait=u32 200) -> ()  [unwired: 1 out]
          }
          frame #2 {
            n176 = global write "Galobal variable_TI.vi" "Rpt Write"(TRUE ("Rework Bit")) -> ()
          }
        }
        n177 = local read "Date time"() -> (w368:string)
        n178 = Select(t="Pass", s=w360, f="Fail") -> (s? t:f=w357:string)
        n179 = Build Array (concatenate)(w368, w367) -> (→"appended array":string[])
        n180 = call "Covert Max &Min data in String.vi"() -> ("out"=w347:T15)  [unwired: 11 in]
        n181 = global read "Galobal variable_TI.vi" "MIC Barcode"() -> (w351:string)
        n182 = Unbundle By Name(w347) -> ("Load Max"=w346:string, "Load Min"=w345:string, "Actuator -1 Max"=w341:string, "Actuator -1 Min"=w340:string, "Actuator -2 Max"=w338:string, "Actuator -2 Min"=w339:string)
        n183 = call "Auotmode.vi"("Enum Selection"=Auot_Test_selection."Enqueue ", "Error In"=w375, "Enqueue"=w370, "queue in"=w376) -> ("error out"=w373:errorcluster, "queue Out"=w374:refnum<queue>)  [unwired: 4 in, 1 out]
        n184 = local read "Actuator1(mm)"() -> (w337:dbl)
        n185 = local read "Actuator2(mm)"() -> (w336:dbl)
        n186 = local read "Load(N)"() -> (w343:dbl)
        n187 = Number To Decimal String(number=w354, width (-)=i16 1) -> (decimal integer string=w353:string)
        n188 = call <vilib>:"Trim Whitespace.vi"("string"=w351, "location (both)"=w349) -> ("trimmed string"=w350:string)
        n189 = Number To Fractional String(number=w337, precision (6)=i16 3 ("width (-)")) -> (F-format string=w332:string)  [unwired: 2 in]
        n190 = Number To Fractional String(number=w336, precision (6)=i16 3 ("width (-)")) -> (F-format string=w333:string)  [unwired: 2 in]
        n191 = Number To Fractional String(number=w343, precision (6)=i16 3 ("width (-)")) -> (F-format string=w342:string)  [unwired: 2 in]
        n192 = global read "Galobal variable_TI.vi" "Lvdt &Load Result"() -> (w348:T9)
        n193 = Bundle By Name(cluster=T11 {"Sr.No."="", "Model Pass/Fail"="", "MIC Code"="", "Clip-1"="", "Clip-2"="", "Clip-3"="", "Clip-4"="", "Load Max"="", "Load Min"="", "Load Actual Value"="", "Actuator -1Min"="", "Actuator -1Max"="", "Actuator-1 Actual Value"="", "Actuator -2Min "="", "Actuator -2Max "="", "Actuator-2 Actual Value "="", "Status"=""} ("Cluster"), "Sr.No."=w353, "Model Pass/Fail"=w357, "MIC Code"=w350, "Clip-1"=w356, "Clip-2"=w356, "Clip-3"=w356, "Clip-4"=w356, "Load Max"=w346, "Load Min"=w345, "Load Actual Value"=w342, "Actuator -1Min"=w340, "Actuator -1Max"=w341, "Actuator-1 Actual Value"=w332, "Actuator -2Min"=w339, "Actuator -2Max"=w338, "Actuator-2 Actual Value"=w333) -> (w331:T11)
        n194 = Unbundle By Name(w348) -> ()  [unwired: 1 out]
        n195 = call "Report data in.vi"("Cluster 2"=w331) -> ("output cluster 4"=w330:T16)  [unwired: 10 in]
        n196 = call "Report Save.vi"("Model No."=w364, "Data In"=w330) -> ()  [unwired: 4 in]
      }
      frame "Error" {
        n197 = call "Pokayoka signal.vi"() -> ("output cluster"=w427:T13)  [unwired: 10 in, 1 out]
        n198 = local write "Cycle Start Bit"(FALSE ("Cycle Start Bit")) -> ()
        n199 = local read "Error  bit"() -> (w419:bool)
        n200 = Unbundle By Name(w427) -> ("Home _3"=w414:bool, "Servo Fault 27"=w422:bool)
        n201 = disable-structure shown="Disabled" {
          disable-tunnel: w414 -> [w496 _]
          frame Disabled {
            w499 = "Safety Error........" ("Error Message")
            n202 = global read "GR_Servo.vi" "Error Message"() -> (w501:string)
            n203 = Equal?(x=w501, y=w499) -> (x = y?=w500:bool)
            n204 = Select(t=w499, s=w500, f="Press Home .........") -> (s? t:f=w497:string)
            n205 = Select(t="Wait for reset", s=w496, f=w497) -> (s? t:f=w502:string)
            n206 = global write "GR_Servo.vi" "Error Message"(w502) -> ()
          }
          frame Enabled {
          }
        }
        n207 = case shown="False" w419 {
          tunnel: [_ w504] -> w413
          frame False {
          }
          frame True {
            n208 = global read "GR_Servo.vi" "Error Message"() -> (w504:string)
            n209 = local write "Error  bit"(FALSE ("Error  bit")) -> ()
            n210 = Concatenate Strings(w504, "." ("string"), "Part NG Press Home PB" ("Error Message")) -> (w508:string)
            n211 = global write "GR_Servo.vi" "Error Message"(w508) -> ()
          }
        }
        n212 = property on="Error Message" class="Str"("Text.BGColor"=u32 16711680, "Blinking"=TRUE) -> ()  [unwired: 2 in, 2 out]
        n213 = call "Tower light.vi"("Enum"=enum16{"Green", "Red", "Yellow"}."Red") -> ()  [unwired: 11 in]
        n214 = Select(t=AutoTest_seq."Cylender Home" ("Enqueue"), s=w414, f=AutoTest_seq."Error" ("Enqueue")) -> (s? t:f=w424:T1)
        n215 = case shown="True" w414 {
          tunnel: w416 -> [_ w525]
          frame False {
          }
          frame True {
            n216 = global read "Galobal variable_TI.vi" "Shift  Change"() -> (w524:string)
            n217 = call "Sub_ shift data reset.vi"("Serial no"="NG Counter.txt" ("File Name"), "Shift"=w524, "Model"=w525) -> ("Serial no"=w527:string)  [unwired: 6 in, 1 out]
            n218 = property on="NG Counter" class="Str"("Value"=w527, "Text.BGColor"=u32 16711680 ("Color Box")) -> ()  [unwired: 2 in, 2 out]
          }
        }
        n219 = case shown="True" w414 {
          tunnel: w416 -> [_ w456]
          frame False {
          }
          frame True {
            n220 = local read "Clip"() -> (w457:T4)
            n221 = flat-sequence {
              tunnel: w457 -> [w482]
              tunnel: w456 -> [w477]
              frame #0 {
                n222 = local read "Actuator2(mm)"() -> (w460:dbl)
                n223 = local read "Actuator1(mm)"() -> (w462:dbl)
                n224 = local read "Load(N)"() -> (w466:dbl)
                n225 = local read "Camera Result"() -> (w479:bool)
                n226 = call "Covert Max &Min data in String.vi"() -> ("out"=w474:T15)  [unwired: 11 in]
                n227 = Cluster To Array(cluster=w482) -> (array=w489:bool[])
                n228 = Number To Fractional String(number=w466, precision (6)=i16 3 ("width (-)")) -> (F-format string=w464:string)  [unwired: 2 in]
                n229 = Number To Fractional String(number=w462, precision (6)=i16 3 ("width (-)")) -> (F-format string=w461:string)  [unwired: 2 in]
                n230 = for {
                  tunnel: w489 -> [w492] mode=indexing
                  tunnel: [w493] -> w488 mode=indexing
                  n231 = Select(t="Pass", s=w492, f="Fail") -> (s? t:f=w493:string)
                }
                n232 = Number To Fractional String(number=w460, precision (6)=i16 3 ("width (-)")) -> (F-format string=w458:string)  [unwired: 2 in]
                n233 = Unbundle By Name(w474) -> ("Load Max"=w473:string, "Load Min"=w472:string, "Actuator -1 Max"=w470:string, "Actuator -1 Min"=w471:string, "Actuator -2 Max"=w468:string, "Actuator -2 Min"=w469:string)
                n234 = Select(t="Pass", s=w479, f="Fail") -> (s? t:f=w478:string)
                n235 = global read "Galobal variable_TI.vi" "MIC Barcode"() -> (w490:string)
                n236 = Array To Cluster(array=w488) -> (cluster=w487:T17)
                n237 = Unbundle By Name(w487) -> ("[0]"=w486:string, "[1]"=w485:string, "[2]"=w484:string, "[3]"=w483:string)
                n238 = Bundle By Name(cluster=T11 {"Sr.No."="", "Model Pass/Fail"="", "MIC Code"="", "Clip-1"="", "Clip-2"="", "Clip-3"="", "Clip-4"="", "Load Max"="", "Load Min"="", "Load Actual Value"="", "Actuator -1Min"="", "Actuator -1Max"="", "Actuator-1 Actual Value"="", "Actuator -2Min "="", "Actuator -2Max "="", "Actuator-2 Actual Value "="", "Status"=""} ("Cluster"), "Model Pass/Fail"=w478, "MIC Code"=w490, "Clip-1"=w486, "Clip-2"=w485, "Clip-3"=w484, "Clip-4"=w483, "Load Max"=w473, "Load Min"=w472, "Load Actual Value"=w464, "Actuator -1Min"=w471, "Actuator -1Max"=w470, "Actuator-1 Actual Value"=w461, "Actuator -2Min"=w469, "Actuator -2Max"=w468, "Actuator-2 Actual Value"=w458, "Status"="Fail") -> (w475:T11)
                n239 = call "Report data in.vi"("Cluster 2"=w475) -> ("output cluster 4"=w491:T16)  [unwired: 10 in]
                n240 = call "Report Save.vi"("Model No."=w477, "Data In"=w491) -> ()  [unwired: 4 in]
              }
            }
          }
        }
        n241 = Not(x=w422) -> (.not. x?=w420:bool)
        n242 = And(x=w414, y=w420) -> (x .and. y?=w421:bool)
        n243 = call "Auotmode.vi"("Enum Selection"=Auot_Test_selection."Enqueue ", "Error In"=w430, "Enqueue"=w424, "queue in"=w432) -> ("error out"=w429:errorcluster, "queue Out"=w431:refnum<queue>)  [unwired: 4 in, 1 out]
        n244 = case shown="True" w421 {
          frame False {
          }
          frame True {
            n245 = for {
              N: 20 -> [_]
              i -> [w515]
              n246 = global read "Galobal variable_TI.vi" "Manual DO"() -> (w512:bool[])
              n247 = Wait (ms)(milliseconds to wait=u32 2) -> ()  [unwired: 1 out]
              n248 = Greater Or Equal?(x=w515, y=10) -> (x >= y?=w513:bool)
              n249 = case shown="False" w513 {
                tunnel: w512 -> [w519 w521]
                tunnel: [w516 w520] -> w511
                frame False {
                  n250 = Replace Array Subset(array=w519, new element=TRUE ("new element/subarray"), index=10) -> (w516:bool[])
                }
                frame True {
                  n251 = Replace Array Subset(array=w521, new element=FALSE ("new element/subarray"), index=10) -> (w520:bool[])
                }
              }
              n252 = global write "Galobal variable_TI.vi" "Manual DO"(w511) -> ()
            }
          }
        }
        n253 = case shown="True" w414 {
          tunnel: w413 -> [_ w437]
          tunnel: w412 -> [w434 w436]
          tunnel: [w434 w435] -> w411
          frame False {
          }
          frame True {
            n254 = stacked-sequence {
              seq-local: [w439 _ _] -> [_ _ w454]
              tunnel: w437 -> [w441 _ _]
              tunnel: w436 -> [w440 _ _]
              tunnel: [_ _ w454] -> w435
              frame #0 {
                n255 = case shown="True" TRUE {
                  tunnel: w441 -> [_ w448]
                  tunnel: w440 -> [w442 w447]
                  tunnel: [w442 w443] -> w439
                  frame False {
                  }
                  frame True {
                    n256 = Increment(x=w447) -> (x+1=w443:u32)
                    n257 = Number To Decimal String(number=w443) -> (decimal integer string=w446:string)  [unwired: 1 in]
                    n258 = Bundle By Name(cluster=T12 {"No. Fail Coun t"="", "Rework Status Count 0\\1"="", "NA Count Max =3 "="", "Testesd Count  0/1"="", "Error code"=""} ("Count For Rework"), "No. Fail Coun t"=w446, "Rework Status Count 0\\1"="1" ("Rework Status Count 0\\1"), "NA Count Max =3"="3", "Testesd Count  0/1"="0", "Error code"=w448) -> (w445:T12)
                    n259 = call "Rework Count.vi"("Read /Write"=enum16{"Write", "Read"}."Write", "Count For Rework"=w445) -> ()  [unwired: 8 in, 2 out]
                  }
                }
              }
              frame #1 {
                n260 = Wait (ms)(milliseconds to wait=u32 200) -> ()  [unwired: 1 out]
              }
              frame #2 {
                n261 = global write "Galobal variable_TI.vi" "Rpt Write"(TRUE ("Rework Bit")) -> ()
              }
            }
          }
        }
      }
      frame "Exit" {
        n262 = global read "Galobal variable_TI.vi" "Manual DO"() -> (w532:bool[])
        n263 = global read "Galobal variable_TI.vi" "Digital input"() -> (w543:bool[])
        n264 = for {
          N: 18 -> [_]
          shift-right: [w552] -> w534
          shift-left: w532 -> [w553]
          i -> [w549]
          stop <- w547 stop-if-true
          n265 = Wait (ms)(milliseconds to wait=u32 50) -> ()  [unwired: 1 out]
          n266 = Greater Or Equal?(x=w549, y=17) -> (x >= y?=w547:bool)
          n267 = Replace Array Subset(array=w553, new element=FALSE ("new element/subarray"), index=w549) -> (w552:bool[])
        }
        n268 = Index Array(array=w543, index #2=1 ("index")) -> (element #2=w533:bool)  [unwired: 1 in, 1 out]
        n269 = local write "Start 2"(T3 FALSE ("Start")) -> ()
        n270 = global write "Galobal variable_TI.vi" "Manual DO"(w534) -> ()
        n271 = Select(t=AutoTest_seq."Poll Event" ("Enqueue"), s=w533, f=AutoTest_seq."Exit" ("Enqueue")) -> (s? t:f=w540:T1)
        n272 = case shown="False" w533 {
          tunnel: [w556 w557] -> w539
          tunnel: w540 -> [w556 w557]
          frame False {
            n273 = call "Tower light.vi"("Enum"=enum16{"Green", "Red", "Yellow"}."Red") -> ()  [unwired: 11 in]
          }
          frame True {
            n274 = call "Tower light.vi"("Enum"=enum16{"Green", "Red", "Yellow"}."Green") -> ()  [unwired: 11 in]
          }
        }
        n275 = global write "GR_Servo.vi" "Error Message"("Relsase  Emergency Pressed" ("Error Message")) -> ()
        n276 = call "Auotmode.vi"("Enum Selection"=Auot_Test_selection."Enqueue ", "Enqueue"=w539, "queue in"=w544) -> ("queue Out"=w545:refnum<queue>)  [unwired: 5 in, 2 out]
        n277 = flat-sequence {
          frame #0 {
            n278 = Wait (ms)(milliseconds to wait=u32 100) -> ()  [unwired: 1 out]
          }
        }
      }
    }
    n279 = global read "Galobal variable_TI.vi" "Auto Exit"() -> (w65:bool)
  }
  n280 = global write "Galobal variable_TI.vi" "Camera NG"(w3) -> ()
  n281 = global write "Galobal variable_TI.vi" "Error color bit"(w3) -> ()
  n282 = global write "Galobal variable_TI.vi" "Camera Ok"(w3) -> ()
  n283 = local write "Start 2"(T3 FALSE ("Start")) -> ()
  n284 = Get Date/Time In Seconds() -> (seconds since 1Jan1904=w33:timestamp)
  n285 = while {
    shift-right: [w595] -> _
    shift-left: w33 -> [w594]
    tunnel: w3 -> [_]
    stop <- w592 stop-if-true
    # "Tracibility"
    n286 = global read "Galobal variable_TI.vi" "Camera NG"() -> (w562:bool)
    n287 = global read "Galobal variable_TI.vi" "Lvdt &Load Result"() -> (w580:T9)
    n288 = global read "Galobal variable_TI.vi" "Error color bit"() -> (w567:bool)
    n289 = global read "Galobal variable_TI.vi" "Camera Ok"() -> (w561:bool)
    "Camera Result" <- w561
    n290 = global read "Galobal variable_TI.vi" "Server"() -> (→"Boolean 3":bool)
    n291 = global read "Galobal variable_TI.vi" "NI Comm.Error"() -> (→"Error":bool)
    n292 = Unbundle By Name(w580) -> ("Actuator1(mm)"=→"Actuator1(mm)":dbl, "Actuator2(mm)"=→"Actuator2(mm)":dbl, "Load(N)"=→"Load(N)":dbl, "Actuator1"=w576:bool, "Actuator2"=w575:bool, "Load"=w574:bool)
    n293 = Get Date/Time In Seconds() -> (seconds since 1Jan1904=w591:timestamp)
    "Current Date & Time" <- w591
    n294 = Select(t=u32 16777226, s=w567, f=u32 16711680) -> (s? t:f=w566:u32)
    n295 = Or(x=w562, y=w561) -> (x .or. y?=w563:bool)
    n296 = property on="Error Message" class="Str"("Text.BGColor"=w566) -> ()  [unwired: 2 in, 2 out]
    n297 = global write "Galobal variable_TI.vi" "Stop M1"(FALSE ("Stop M1")) -> ()
    n298 = Build Array(w576, w575, w574) -> (w573:bool[])
    n299 = case shown="False" "Cycle Start Bit" {
      tunnel: w594 -> [_ w602]
      tunnel: w591 -> [w600 w603]
      tunnel: [w600 w602] -> w595
      frame False {
      }
      frame True {
        n300 = Subtract(x=w603, y=w602) -> (x-y=w604:dbl)
        n301 = To Long Integer(number=w604) -> (32bit integer=w601:i32)
        "Cycle Time(Sec)" <- w601
        n302 = local write "Cycle"(w601) -> ()
      }
    }
    n303 = property on="Camera Result" class="Bool (strict)"("Visible"=w563) -> ()  [unwired: 2 in, 2 out]
    n304 = for {
      tunnel: w573 -> [w599] mode=indexing
      tunnel: [w596] -> w572 mode=indexing
      n305 = Select(t=u32 4390733, s=w599, f=u32 16711680) -> (s? t:f=w596:u32)
    }
    n306 = global read "Galobal variable_TI.vi" "Auto Exit"() -> (w592:bool)
    n307 = Get Date/Time In Seconds() -> (seconds since 1Jan1904=w588:timestamp)
    n308 = global read "Galobal variable_TI.vi" "Running Model"() -> (→"Running Model":string)
    n309 = global read "Galobal variable_TI.vi" "MIC Barcode"() -> (→"PCB Barcode":string)
    n310 = Index Array(array=w572) -> (element #1=w571:u32, element #2=w570:u32, element #3=w569:u32)  [unwired: 3 in]
    n311 = Select(t=enum32{"Test", "Report"}."Report" ("Tab Control"), s="Report", f=enum32{"Test", "Report"}."Test" ("Tab Control")) -> (s? t:f=w582:enum32{"Test", "Report"})
    n312 = property on="Actuator1(mm)" class="DigNum (strict)"("NumText.BGColor"=w571) -> ()  [unwired: 2 in, 2 out]
    n313 = property on="Actuator2(mm)" class="DigNum (strict)"("NumText.BGColor"=w570) -> ()  [unwired: 2 in, 2 out]
    n314 = property on="Load(N)" class="DigNum (strict)"("NumText.BGColor"=w569) -> ()  [unwired: 2 in, 2 out]
    n315 = Format Date/Time String(time format string (%c)="%d-%m-%Y  %H:%M:%S", seconds (now)=w588) -> (date/time string=→"Date time":string)  [unwired: 1 in]
    n316 = global write "Galobal variable_TI.vi" "Tracibility"("Boolean") -> ()
    n317 = local write "Tab Control"(w582) -> ()
  }
  n318 = while {
    stop <- w606 stop-if-true
    n319 = event shown="[0] Timeout" {
      selector: _ -> [_ _ _]
      dyn-events: _ -> [_ _ _]
      timeout: 2 -> [_ _ _]
      event Timeout {
        n320 = event-data() -> ()  [unwired: 1 in, 3 out]
        n321 = global read "GR_Servo.vi" "Error Message"() -> (→"Error Message":string)
        n322 = global read "Galobal variable_TI.vi" "Digital input"() -> (w623:bool[])
        n323 = global read "Galobal variable_TI.vi" "Digital input"() -> (w631:bool[])
        n324 = Index Array(array=w623, index #1=20 ("index"), index #2=21 ("index"), index #3=22 ("index"), index #4=23 ("index"), index #5=16 ("index"), index #6=17 ("index"), index #7=27 ("index")) -> (element #1=w611:bool, element #2=w610:bool, element #3=w609:bool, element #4=w608:bool, element #7=→"Servo Fault":bool)  [unwired: 2 out]
        n325 = Bundle By Name(cluster=T4 {"Cllip-3 (AI12)"=FALSE, "Cllip-4 (AI9)"=FALSE, "Cllip-2(AI10)"=FALSE, "Cllip-1 (AI9)"=FALSE} ("Clip 2"), "Cllip-1 (AI9)"=w611, "Cllip-2(AI10)"=w610, "Cllip-3 (AI12)"=w609, "Cllip-4 (AI9)"=w608) -> (→"Clip":T4)
        n326 = Index Array(array=w631, index #1=0 ("index"), index #2=8 ("index"), index #3=2 ("index")) -> (element #1=→"Start":bool, element #2=w627:bool, element #3=→"reset":bool)
        n327 = global read "Galobal variable_TI.vi" "STM Done Bit"() -> (w628:bool)
        n328 = Or(x=w627, y=w628) -> (x .or. y?=w626:bool)
        n329 = Select(t=cluster{u32, u32}[] [{16734762, 6618880}, {16777222, 6618880}] ("Colors [4]"), s=w626, f=cluster{u32, u32}[] [{16734762, 16711680}, {16777222, 16775560}] ("Colors [4]")) -> (s? t:f=w632:cluster{u32, u32}[])
        n330 = property on="Slide Servo Home Call" class="Bool (strict)"("Colors [4]"=w632) -> ()  [unwired: 2 in, 2 out]
      }
      event "Servo Fault Reset": Value Change {
        n331 = event-data() -> ("NewVal"=w635:bool)  [unwired: 1 in]
        n332 = global read "Galobal variable_TI.vi" "Manual DO"() -> (w638:bool[])
        n333 = Replace Array Subset(array=w638, new element=w635, index=1) -> (w637:bool[])
        n334 = global write "Galobal variable_TI.vi" "Manual DO"(w637) -> ()
      }
      event Value Change {
        n335 = event-data() -> ("NewVal"=w639:T2)  [unwired: 1 in]
        n336 = global write "Galobal variable_TI.vi" "Auto Exit"(w639) -> ()
        n337 = global read "Galobal variable_TI.vi" "Digital input"() -> (→"DI":bool[])
      }
    }
    n338 = local read "Exit"() -> (w606:T2)
  }
  n339 = call "Auotmode.vi"("Enum Selection"=Auot_Test_selection."Flush", "Error In"=w28, "queue in"=w34) -> ("error out"=w39:errorcluster, "queue Out"=w38:refnum<queue>)  [unwired: 5 in, 1 out]
  n340 = call "Auotmode.vi"("Enum Selection"=Auot_Test_selection."Release Queue", "Error In"=w39, "queue in"=w38) -> ("error out"=→"error out":errorcluster)  [unwired: 5 in, 2 out]
